vi "mupPostInstall.vi"   [LabVIEW 2018]
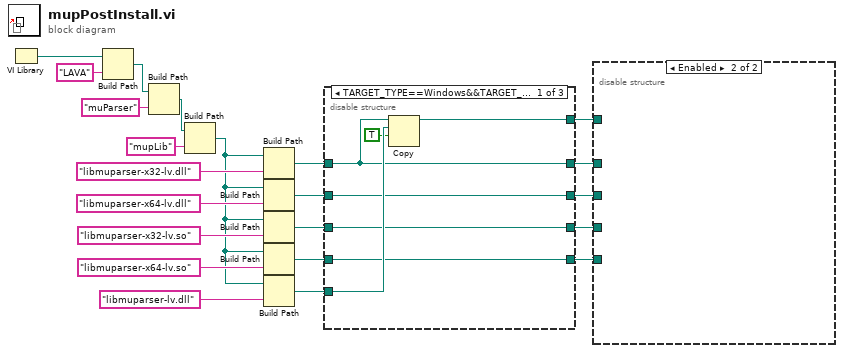
[diagram p0: block diagram]
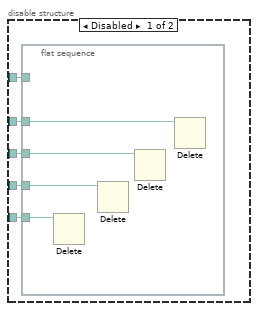
[diagram p2: hidden frame]
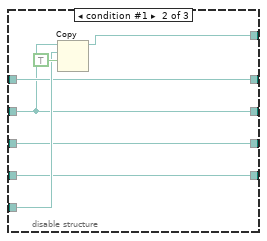
[diagram p3: hidden frame]
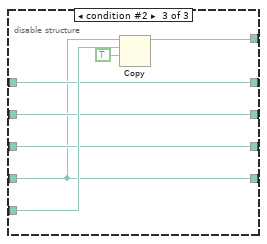
[diagram p4: hidden frame]
diagram:
  n1 = VI Library() -> (path=w6:path)
  n2 = Build Path(base path=w6, name or relative path="LAVA") -> (appended path=w5:path)
  n3 = Build Path(base path=w5, name or relative path="muParser") -> (appended path=w2:path)
  n4 = Build Path(base path=w2, name or relative path="mupLib") -> (appended path=w1:path)
  n5 = Build Path(base path=w1, name or relative path="libmuparser-x32-lv.dll") -> (appended path=w17:path)
  n6 = Build Path(base path=w1, name or relative path="libmuparser-x64-lv.dll") -> (appended path=w14:path)
  n7 = Build Path(base path=w1, name or relative path="libmuparser-x32-lv.so") -> (appended path=w13:path)
  n8 = Build Path(base path=w1, name or relative path="libmuparser-x64-lv.so") -> (appended path=w12:path)
  n9 = Build Path(base path=w1, name or relative path="libmuparser-lv.dll") -> (appended path=w15:path)
  n10 = disable-structure shown="TARGET_TYPE==Windows&&TARGET_BITNESS==32||OS==Win&&TARGET_BITNESS==32, Default" {
    disable-tunnel: w17 -> [w27 w34 w41]
    disable-tunnel: w15 -> [w29 w35 w42]
    disable-tunnel: w14 -> [w26 w33 w40]
    disable-tunnel: w13 -> [w25 w32 w39]
    disable-tunnel: w12 -> [w24 w31 w38]
    disable-tunnel: [w27 w34 w41] -> w10
    disable-tunnel: [w26 w33 w40] -> w9
    disable-tunnel: [w25 w32 w39] -> w8
    disable-tunnel: [w24 w31 w38] -> w7
    disable-tunnel: [w23 w30 w37] -> w11
    frame condition #0 (active) {
      n11 = Copy(9:TRUE ("overwrite (F)"), 10:w29, 11:w27) -> (3:w23:path)  [unwired: 2 in, 2 out]
    }
    frame condition #1 {
      n12 = Copy(9:TRUE ("overwrite (F)"), 10:w35, 11:w33) -> (3:w30:path)  [unwired: 2 in, 2 out]
    }
    frame condition #2 {
      n13 = Copy(9:TRUE ("overwrite (F)"), 10:w42, 11:w38) -> (3:w37:path)  [unwired: 2 in, 2 out]
    }
  }
  n14 = disable-structure shown="Enabled" {
    disable-tunnel: w11 -> [w48 _]
    disable-tunnel: w10 -> [w47 _]
    disable-tunnel: w9 -> [w46 _]
    disable-tunnel: w8 -> [w45 _]
    disable-tunnel: w7 -> [w44 _]
    frame Disabled {
      n15 = flat-sequence {
        tunnel: w48 -> [_]
        tunnel: w47 -> [w52]
        tunnel: w46 -> [w51]
        tunnel: w45 -> [w50]
        tunnel: w44 -> [w49]
        frame #0 {
          n16 = Delete(path (use dialog)=w49) -> ()  [unwired: 4 in, 3 out]
          n17 = Delete(path (use dialog)=w50) -> ()  [unwired: 4 in, 3 out]
          n18 = Delete(path (use dialog)=w51) -> ()  [unwired: 4 in, 3 out]
          n19 = Delete(path (use dialog)=w52) -> ()  [unwired: 4 in, 3 out]
        }
      }
    }
    frame Enabled {
    }
  }
